vi "MainConvertiMisure_INPUT.vi"(11 "Array Misure Input":dbl[](array[numeric])) -> (3 "Array Misure/Unità OUT":T1[](array[typedef]))   [LabVIEW 2016]
uses:
  <vilib>/Utility/file.llb/Read Delimited Spreadsheet (string).vi
panel:
  in  "Cluster Misura / Unità":T1
  out "Caratteristiche Caricate":string[][](array[string])
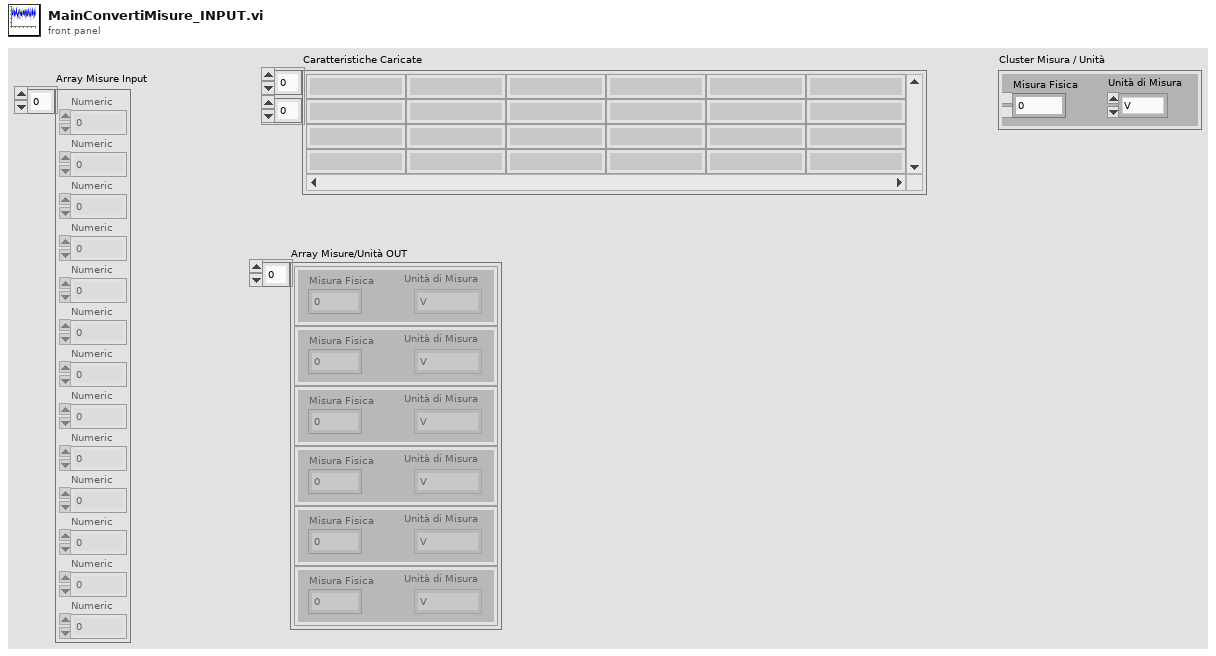
[diagram p1: front panel]
types:
  T1 = typedef "ClusterMisura_e_Unità_INPUT.ctl" = cluster{"Misura Fisica":dbl, "Unità di Misura":T2}
  T2 = typedef "UnitàMisura.ctl" = enum16{"V", "mA", "Bar", "RPM", "m3/s", "m3/min", "m3/h", "l/s", "l/min", "in3/min", "ft3/min", "gpm", "igpm", "igph"}
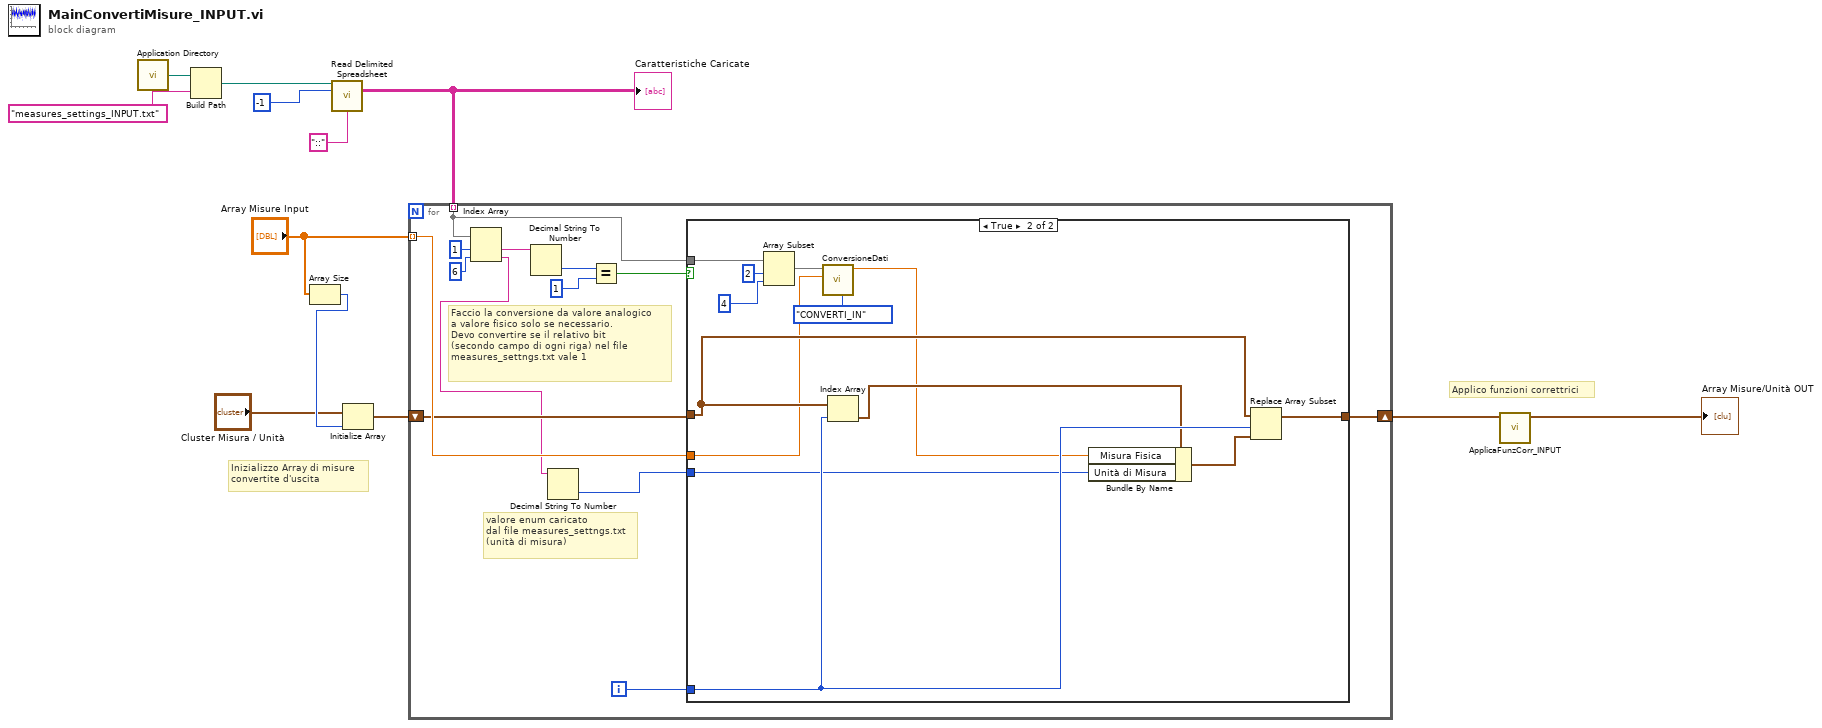
[diagram p0: block diagram]
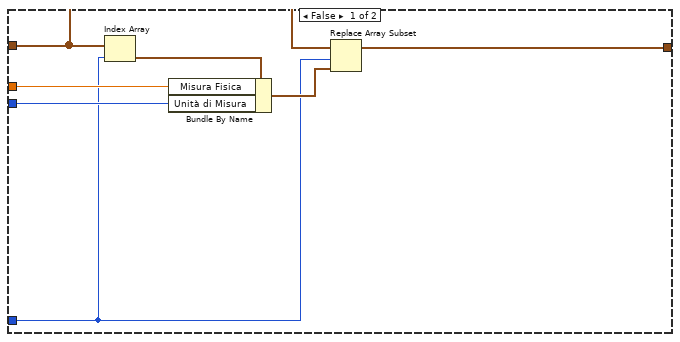
[diagram p2: hidden frame]
diagram:
  # "Applico funzioni correttrici"
  # "Inizializzo Array di misure \nconvertite d'uscita"
  n1 = call <vilib>:"Application Directory.vi"() -> ("Application Directory"=w11:path)
  n2 = Build Path(base path=w11, name or relative path="measures_settings_INPUT.txt") -> (appended path=w10:path)
  n3 = Array Size(array="Array Misure Input") -> (size(s)=w5:i32)
  n4 = call-poly <vilib>:"Read Delimited Spreadsheet.vi"("file path (dialog if empty)"=w10, "number of rows (all:-1)"=-1, "delimiter (\\t)"="::" ("delimiter (\\t)")) -> ("all rows"=w7:string[][])  [unwired: 7 in, 5 out]
  "Caratteristiche Caricate" <- w7
  n5 = Initialize Array("Cluster Misura / Unità", w5) -> (w4:T1[])
  n6 = for {
    tunnel: "Array Misure Input" -> [w20] mode=indexing
    tunnel: w7 -> [w14] mode=indexing
    shift-right: [w15] -> w2
    shift-left: w4 -> [w19]
    i -> [w13]
    # "valore enum caricato\ndal file measures_settngs.txt \n(unità di misura)"
    # "Faccio la conversione da valore analogico\na valore fisico solo se necessario. \nDevo convertire se il relativo bit \n(secondo campo di ogni riga) nel file \nmeasures_settngs.txt vale 1"
    n7 = Index Array(array=w14, index #1=1 ("index"), index #2=6 ("index")) -> (element #1=w24:string, element #2=w17:string)
    n8 = Decimal String To Number(string=w24) -> (number=w23:i32)  [unwired: 2 in, 1 out]
    n9 = Decimal String To Number(string=w17) -> (number=w16:i32)  [unwired: 2 in, 1 out]
    n10 = Equal?(x=w23, y=1) -> (x = y?=w21:bool)
    n11 = case shown="True" w21 {
      tunnel: w20 -> [w31 w37]
      tunnel: w19 -> [w28 w42]
      tunnel: w13 -> [w27 w44]
      tunnel: w16 -> [w30 w40]
      tunnel: [w26 w41] -> w15
      tunnel: w14 -> [_ w39]
      frame False {
        n12 = Index Array(array=w28, index=w27) -> (element=w32:T1)
        n13 = Bundle By Name(cluster=w32, "Misura Fisica"=w31, "Unità di Misura"=w30) -> (w29:T1)
        n14 = Replace Array Subset(array=w28, new element=w29, index=w27) -> (w26:T1[])
      }
      frame True {
        n15 = Array Subset(array=w39, index=2, length=4 ("index")) -> (w38:string[])
        n16 = call "ConversioneDati.vi"("Stato Conversione"=enum16{"CONVERTI_IN", "CONVERTI_OUT"}."CONVERTI_IN", "Data"=w37, "Impostazioni Conversione"=w38) -> ("Dato Convertito"=w36:dbl)  [unwired: 8 in]
        n17 = Index Array(array=w42, index=w44) -> (element=w43:T1)
        n18 = Bundle By Name(cluster=w43, "Misura Fisica"=w36, "Unità di Misura"=w40) -> (w45:T1)
        n19 = Replace Array Subset(array=w42, new element=w45, index=w44) -> (w41:T1[])
      }
    }
  }
  n20 = call "ApplicaFunzCorr_INPUT.vi"("Array"=w2) -> ("Array Cluster Corretto"=→"Array Misure/Unità OUT":T1[])  [unwired: 9 in]
